vi "CLD 14 FGV Timer.vi"(8 "Fehler (Eingang)":T1, 10 "Zielzeit (s) [0]":dbl, 11 "CLD 14 - FGV-Enum":T2) -> (0 "Fehler (Ausgang)":T1, 1 "Zielzeit (Ausgang)":dbl, 2 "Ist Zeit verstrichen?":bool, 3 "Verstrichene Zeit (s,ms)":dbl format="%#_2g", 4 "Anhalten?":bool)   [LabVIEW 2009]
doc: "CLD-Übung 14\nDieses VI wird als FGV verwendet. \nHinweis zum Auslesen der Zeit während der Pause. Der Entwickler sollte die Funktion \"Zeit lesen\" nicht während der Pause aufrufen. Mit Hilfe einer Case-Struktur kann \"Status abfragen\" jedoch präventiv für diese Möglichkeit programmiert werden."
uses:
  CLD 14 FGV Enum.ctl
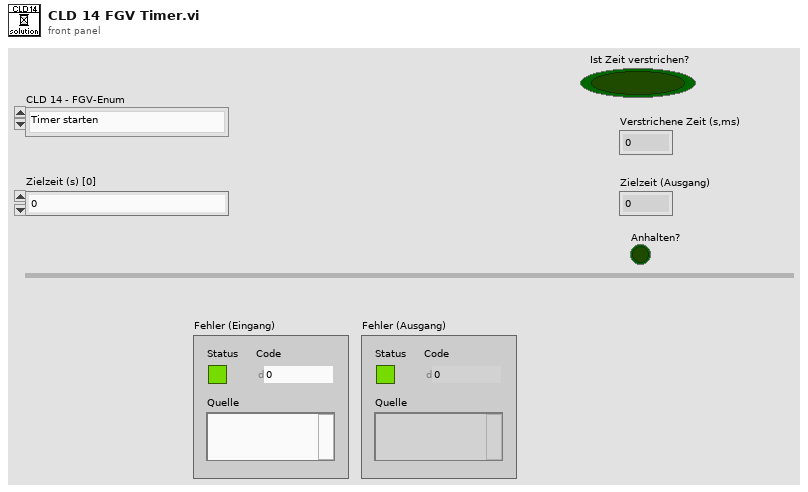
[diagram p1: front panel]
types:
  T1 = cluster{"Status":bool, "Code":i32, "Quelle":string}
  T2 = typedef "CLD 14 FGV Enum.ctl" = enum16{"Timer starten", "Zeit lesen", "Anhalten", "Fortsetzen"}
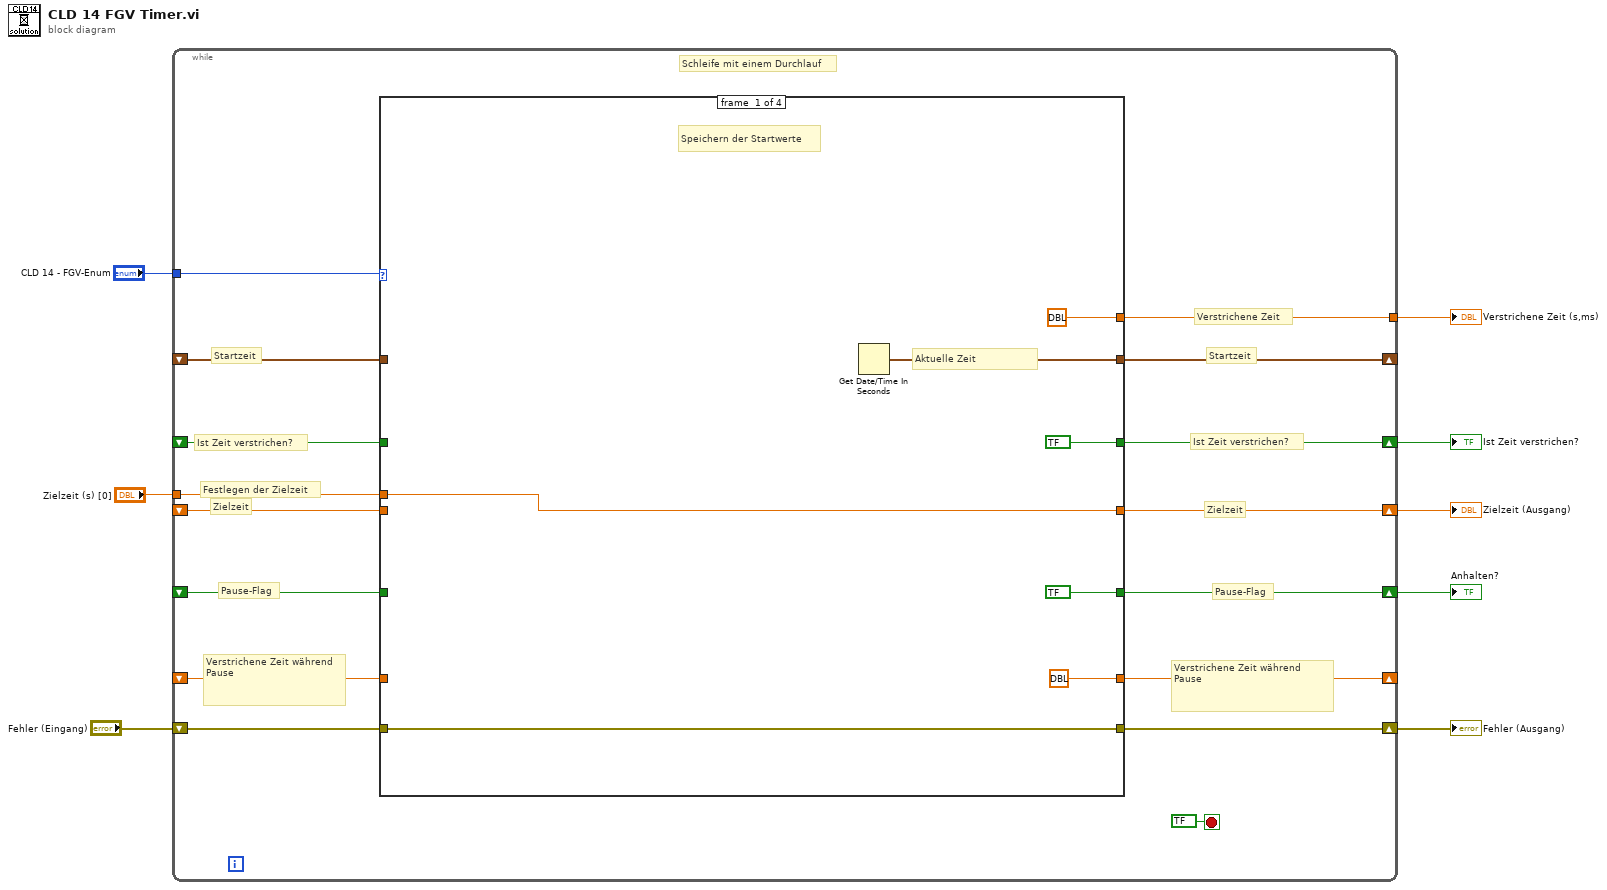
[diagram p0: block diagram]
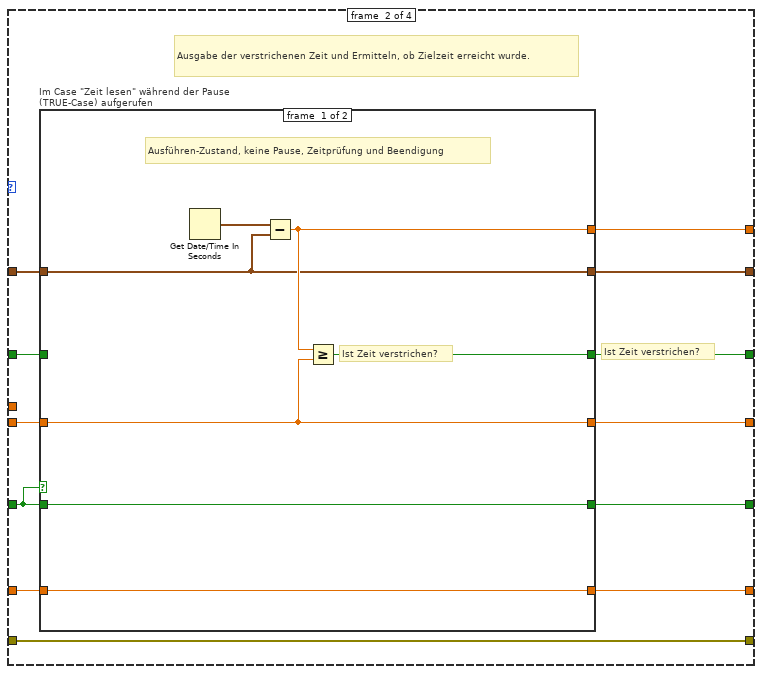
[diagram p2: hidden frame]
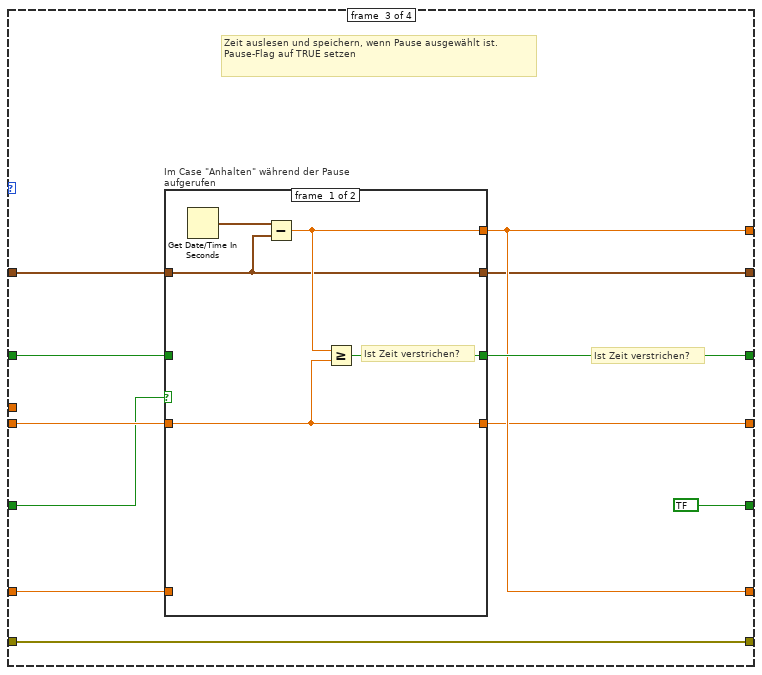
[diagram p4: hidden frame]
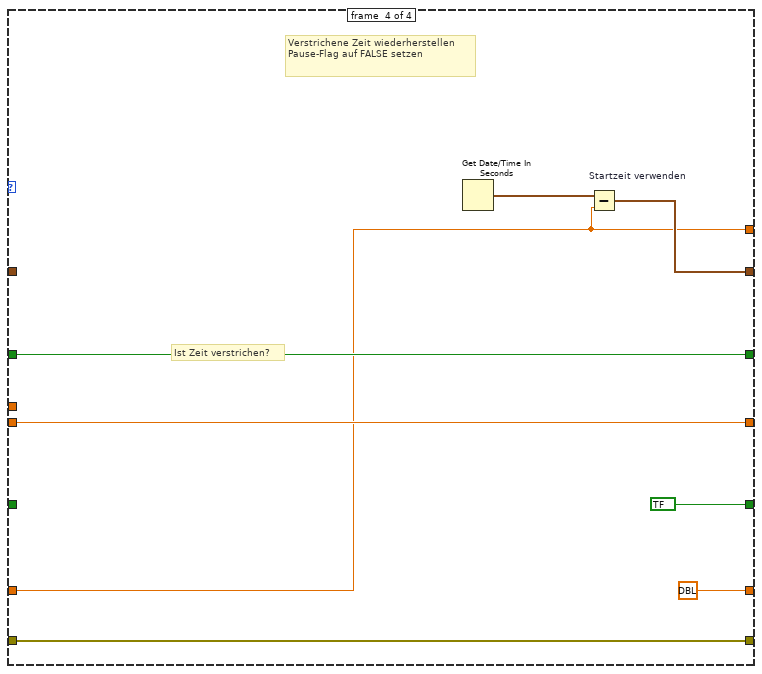
[diagram p6: hidden frame]
diagram:
  n1 = while {
    tunnel: "CLD 14 - FGV-Enum" -> [w24]
    shift-right: [w22] -> _
    shift-left: _ -> [w21]
    tunnel: [w20] -> w1
    shift-right: [w19] -> w7
    shift-left: "Fehler (Eingang)" -> [w18]
    tunnel: "Zielzeit (s) [0]" -> [w15]
    shift-right: [w16] -> w3
    shift-left: _ -> [w17]
    shift-right: [w14] -> w4
    shift-left: _ -> [w13]
    shift-right: [w12] -> w2
    shift-left: _ -> [w11]
    shift-right: [w10] -> _
    shift-left: _ -> [w9]
    stop <- bool ? ("Stopp") stop-if-true
    # "Startzeit"
    # "Startzeit"
    # "Verstrichene Zeit"
    # "Zielzeit"
    # "Zielzeit"
    # "Festlegen der Zielzeit"
    # "Ist Zeit verstrichen?"
    # "Ist Zeit verstrichen?"
    # "Pause-Flag"
    # "Pause-Flag"
    # "Verstrichene Zeit während Pause"
    # "Verstrichene Zeit während Pause"
    # "Schleife mit einem Durchlauf"
    n2 = case shown="\"Zeit lesen\"" w24 {
      tunnel: [w31 w37 w56 w77] -> w22
      tunnel: w21 -> [_ w43 w66 _]
      tunnel: [dbl ? ("Verstrichene Zeit") w40 w61 w76] -> w20
      tunnel: [w29 w42 w65 w83] -> w19
      tunnel: w18 -> [w29 w42 w65 w83]
      tunnel: w17 -> [_ w32 w64 w82]
      tunnel: [w28 w33 w57 w82] -> w16
      tunnel: w15 -> [w28 _ _ _]
      tunnel: [bool ? w41 w63 w80] -> w14
      tunnel: w13 -> [_ w34 w60 w80]
      tunnel: [bool ? w36 bool ? bool ?] -> w12
      tunnel: w11 -> [_ w35 w59 _]
      tunnel: [dbl ? w38 w61 dbl ?] -> w10
      tunnel: w9 -> [_ w39 w58 w76]
      frame #0 {
        # "Aktuelle Zeit"
        # "Speichern der Startwerte"
        n3 = Get Date/Time In Seconds() -> (seconds since 1Jan1904=w31:timestamp)
      }
      frame #1 {
        # "Ist Zeit verstrichen?"
        # "Ausgabe der verstrichenen Zeit und Ermitteln, ob Zielzeit erreicht wurde."
        n4 = case "Im Case \"Zeit lesen\" während der Pause (TRUE-Case) aufgerufen" shown="True" w35 {
          tunnel: w43 -> [w47 w55]
          tunnel: w32 -> [w46 w54]
          tunnel: [w49 w52] -> w41
          tunnel: [w48 w51] -> w40
          tunnel: w39 -> [w44 w51]
          tunnel: [w44 w51] -> w38
          tunnel: [w47 w55] -> w37
          tunnel: [w46 w54] -> w33
          tunnel: [w45 w53] -> w36
          tunnel: w35 -> [w45 w53]
          tunnel: w34 -> [_ w52]
          frame #0 {
            # "Ist Zeit verstrichen?"
            # "Ausführen-Zustand, keine Pause, Zeitprüfung und Beendigung"
            n5 = Get Date/Time In Seconds() -> (seconds since 1Jan1904=w50:timestamp)
            n6 = Subtract(x=w50, y=w47) -> (x-y=w48:dbl)
            n7 = Greater Or Equal?(x=w48, y=w46) -> (x >= y?=w49:bool)
          }
          frame #1 {
            # "Pause-Zustand, nur Ausgabe von Schieberegistern. \"Zeit lesen\" nicht während der Pause aufrufen."
          }
        }
      }
      frame #2 {
        # "Ist Zeit verstrichen?"
        # "Zeit auslesen und speichern, wenn Pause ausgewählt ist.\nPause-Flag auf TRUE setzen"
        n8 = case "Im Case \"Anhalten\" während der Pause aufgerufen" shown="True" w59 {
          tunnel: w66 -> [w67 w72]
          tunnel: w64 -> [w68 w73]
          tunnel: [w70 w75] -> w63
          tunnel: [w69 w74] -> w61
          tunnel: w60 -> [_ w75]
          tunnel: w58 -> [_ w74]
          tunnel: [w68 w73] -> w57
          tunnel: [w67 w72] -> w56
          frame #0 {
            # "Ist Zeit verstrichen?"
            n9 = Get Date/Time In Seconds() -> (seconds since 1Jan1904=w71:timestamp)
            n10 = Subtract(x=w71, y=w67) -> (x-y=w69:dbl)
            n11 = Greater Or Equal?(x=w69, y=w68) -> (x >= y?=w70:bool)
          }
          frame #1 {
            # "Pause wurde während der Pause aufgerufen.\n\nNur Schieberegister auslesen und Werte weitergeben."
          }
        }
      }
      frame #3 {
        # "Ist Zeit verstrichen?"
        # "Verstrichene Zeit wiederherstellen\nPause-Flag auf FALSE setzen"
        n12 = Get Date/Time In Seconds() -> (seconds since 1Jan1904=w78:timestamp)
        n13 = Subtract "Startzeit verwenden"(x=w78, y=w76) -> (x-y=w77:timestamp)
      }
    }
  }
  "Fehler (Ausgang)" <- w7
  "Ist Zeit verstrichen?" <- w4
  "Verstrichene Zeit (s,ms)" <- w1
  "Zielzeit (Ausgang)" <- w3
  "Anhalten?" <- w2
